vi "RFH-utility-get_all_paths.vi"(7 "Folder Path":path, 8 "error in (no error)":errorcluster, 9 "pattern":string) -> (0 "error out":errorcluster, 1 "All Files in Dir":path[](array[path]), 2 "All Folders":path[](array[path]), 4 "empty?":bool)   [LabVIEW 2020, in "RFH-Reflection_File_Handler.lvlib"]
uses:
  RFH-Reflection_File_Handler.lvlib
panel:
  out "array w/ subset deleted":path[](array[path])
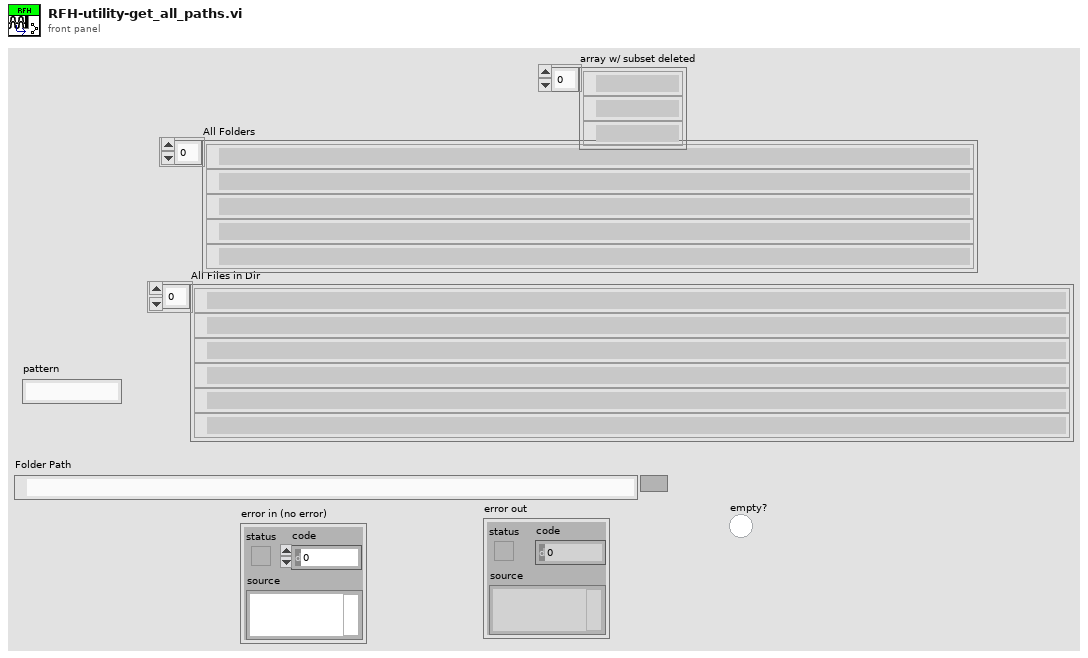
[diagram p1: front panel]
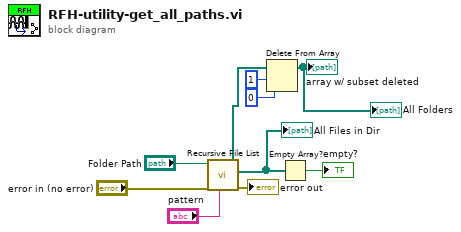
[diagram p0: block diagram]
diagram:
  n1 = call <vilib>:"Recursive File List.vi"("pattern"="pattern", "error in (no error)"="error in (no error)", "Folder Path"="Folder Path") -> ("error out"=→"error out":errorcluster, "All Files in Dir"=w7:path[], "All Folders"=w2:path[])  [unwired: 4 in, 2 out]
  "All Files in Dir" <- w7
  n2 = Delete From Array(array=w2, length=1, index=0) -> (array with subset deleted=→"All Folders" →"array w/ subset deleted":path[])  [unwired: 1 out]
  n3 = Empty Array?(array=w7) -> (empty?=→"empty?":bool)
